vi "HB Timeout.vi"(10 "HB Timeout ms":u32=5000) -> (2 "Timeout":bool, 3 "millisecond timer value":u32)   [LabVIEW 2018, in "MQTT_Singleton.lvlib"]
uses:
  MQTT_Singleton.lvlib
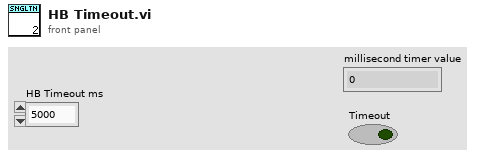
[diagram p1: front panel]
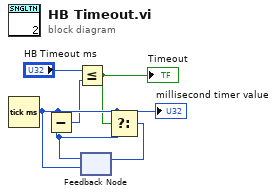
[diagram p0: block diagram]
diagram:
  n1 = Tick Count (ms)() -> (millisecond timer value=w6:u32)
  "millisecond timer value" <- w6
  n2 = feedback #1(w6) -> (w2:u32)
  n3 = Subtract(x=w6, y=w2) -> (x-y=w3:u32)
  n4 = Less Or Equal?(x="HB Timeout ms", y=w3) -> (x <= y?=w5:bool)
  "Timeout" <- w5
  n5 = Select(t=w6, s=w5, f=w2) -> (s? t:f=w1:u32)
  n6 = feedback-in #1(w1) -> ()
